vi "Read Init.vi"(8 "error in (no error)":errorcluster, 11 "Toggle 8 in":refnum<class "Toggle 8.lvclass">) -> (0 "error out":errorcluster, 2 "Init":T1[](array[typedef])=[{"Register"=0, "Value"=0, "Dev Address"=7, "Physical Adress"=0}, {"Register"=0, "Value"=128, "Dev Address"=7, "Physical Adress"=0}], 3 "Toggle 8 out":refnum<class "Toggle 8.lvclass">)   [LabVIEW 2020, in "Toggle 8.lvclass"]
uses:
  Toggle 8.lvclass
  Controls/Register to Write.ctl
  Toggle 8.lvclass/Toggle 8.ctl
  PIC-device/PIC-Device.lvclass
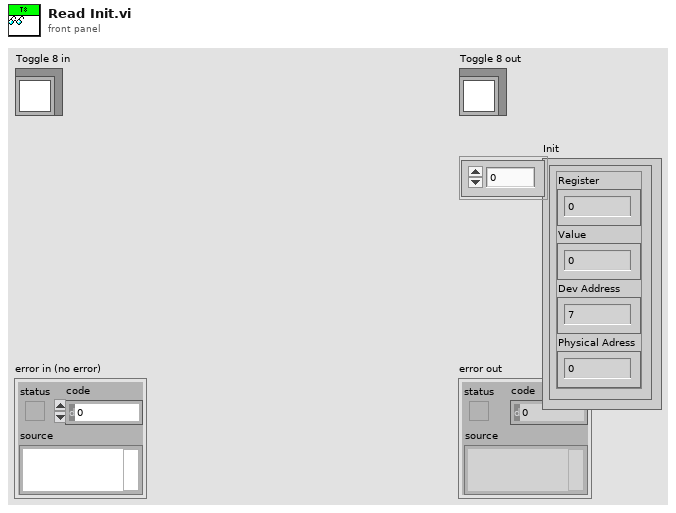
[diagram p1: front panel]
types:
  T1 = typedef "PIC-Device.lvclass/Register to Write.ctl" = cluster{"Register":u32, "Value":u32, "Dev Address":u32, "Physical Adress":u32}
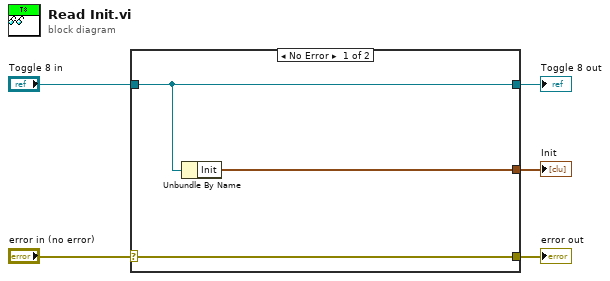
[diagram p0: block diagram]
diagram:
  n1 = case shown="No Error" "error in (no error)" {
    selector: "error in (no error)" -> [w8 w9]
    tunnel: [w8 w9] -> w4
    tunnel: [w7 w10] -> w2
    tunnel: "Toggle 8 in" -> [w7 w10]
    tunnel: [w6 _] -> w1
    frame No Error {
      n2 = Unbundle By Name(w7) -> ("Init"=w6:T1[])
    }
    frame Error {
    }
  }
  "error out" <- w4
  "Toggle 8 out" <- w2
  "Init" <- w1
